vi "Classifier Utility.vi"() -> ()   [LabVIEW 2016]
uses:
  <vilib>/vision/Classification.llb/IMAQ SVM Kernel Options.ctl
  _vlib/CU_ClassifierQualityMeasure.ctl
  _vlib/CU_metaParameters.ctl
  _vlib/CU_metaIndicators.ctl
  Classifier.lvlib
  <vilib>/Analysis/NI_AALBase.lvlib
panel:
  in  "Stop Button":bool
  in  "Tab Control":T1(tab)
  in  "ClassifierQualityMeasure":T2 caption="Критерий оценки точности классификации"
  in  "Training data paths":path[](array[path]) caption="Пути к файлам с обучающими данными"
  in  "Test data paths":path[](array[path]) caption="Пути к файлам с тестовыми данными"
  in  "True labels for Test data":path[](array[path]) caption="Пути к файлам с метками классов (для тестовых данных)"
  in  "Start GA":bool
  in  "SVM ClassifierOptions":T3={"Kernel"=enum."Linear", "Degree"=3, "Gamma"=1.0, "Coefficient"=0.0, "Sigma"=1.0, "Cache(MB)"=200.0} caption="Настройки метода опорных векторов"
  in  "Pointer Slide":dbl(slide) caption="Сократить число признаков на %" min=0.0 max=100.0 step=1.0 scale=0.0..100.0
  in  "Use equal number of trials?":bool caption="Включить балансировку классов?"
  out "kNN accuracy":dbl caption="Макс. среднее\nзнач. точности"
  out "Best k value":dbl caption="Оптимальное\nзначение k"
  out "kNN classifier":cluster{dbl[], dbl[]}[](graph) caption="Метод k ближайших соседей"
  out "SVM classifier":cluster{dbl[], dbl[]}[](graph) caption="Метод опорных векторов"
  out "Best Nu value":dbl caption="Оптимальное \nзначение Nu"
  out "SVM accuracy":dbl caption="Макс. среднее\nзнач. точности"
  out "MLP accuracy":dbl caption="Макс. среднее\nзнач. точности"
  out "Best N value":dbl caption="Оптимальное\nзначение N"
  out "MLP classifier":cluster{dbl[], dbl[]}[](graph) caption="Многослойный персептрон"
  out "Dataset Num":i32
  out "Total Progress":i32(slide) scale=0.0..3.0
  out "Solution":i32(listbox) caption="Оценки точности классификации"
  out "Accuracies Graph":cluster{dbl[], dbl[]}[](graph) caption="Графики точности классификации"
  out "Results":string caption="Протокол выполнения программы"
  out "Accuracies out":dbl[][](array[numeric]) caption="Оценки точности классификации" format="%#_3g"
  out "Average  Accuracies":dbl[][](array[numeric]) caption="Точность классификации по всем наборам данных" format="%#_3g"
  # "This VI is a part of BCI Design library, http://www.ru-bci.org \nCopyright © 2020, Sotnikov Peter, All rights reserved. License: GNU GPLv3"
  # "Общее выполнение"
  # "Набор данных №"
  # "Выбор оптимальных параметров классификаторов"
  # "Методы классификации"
  # "Среднее\nпо наборам"
  # "Метод классификации"
  # "K1"
  # "K2"
  # "K3"
  # "K4"
  # "K5"
  # "Среднее значение"
  # "Среднеквадратич. отклонение"
  # "Максимальное значение"
  # "Минимальное значение"
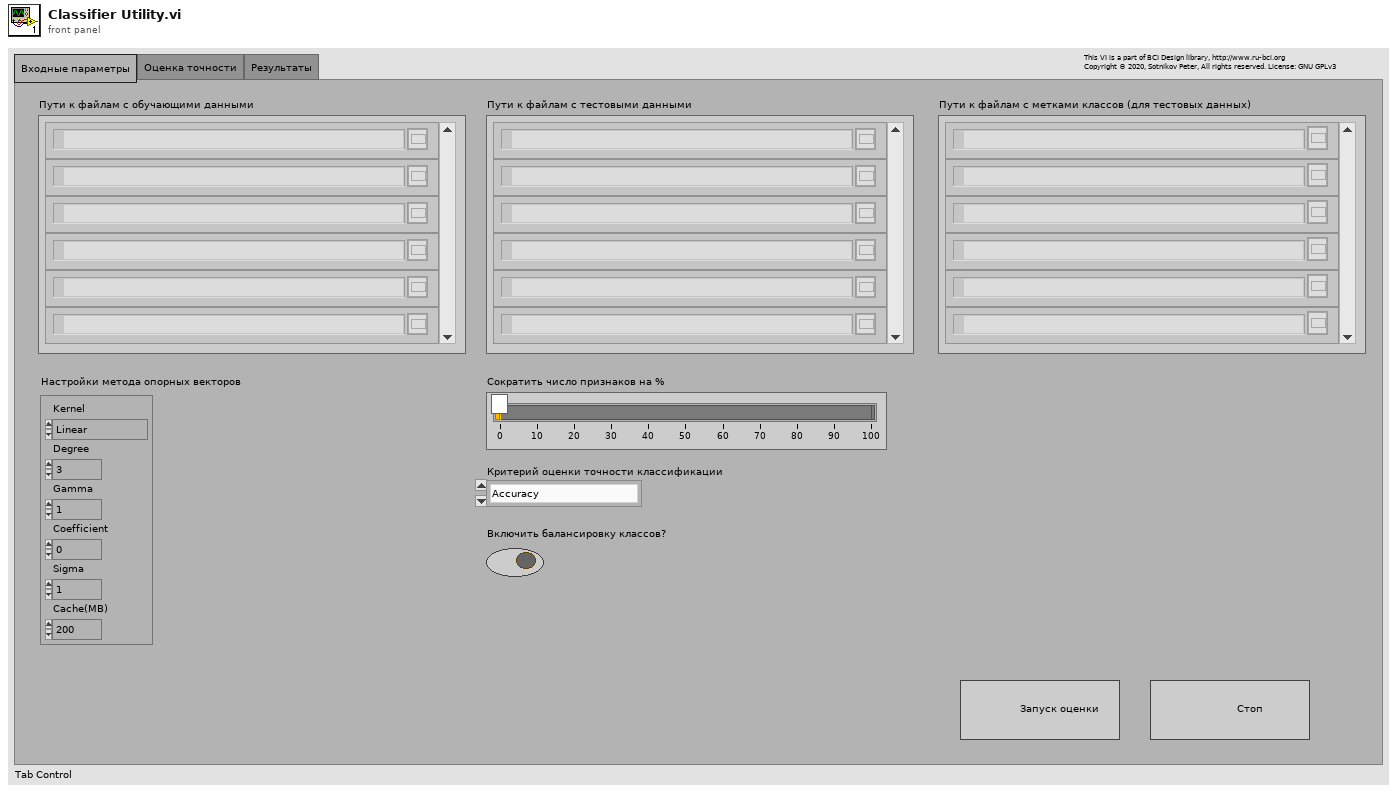
[diagram p1: front panel]
types:
  T1 = enum32{"Входные параметры", "Оценка точности", "Результаты"}
  T2 = typedef "Classifier.lvlib/CU_ClassifierQualityMeasure.ctl" = enum16{"Accuracy", "Cohen's kappa"}
  T3 = typedef "IMAQ SVM Kernel Options.ctl" = cluster{"Kernel":enum32{"Linear", "Polynomial", "Gaussian", "RBF"}, "Degree":i32, "Gamma":dbl, "Coefficient":dbl, "Sigma":dbl, "Cache(MB)":dbl}
  T4 = typedef "Classifier.lvlib/CU_metaIndicators.ctl" = cluster{"Accuracy Charts":refnum<vi>[], "Best Parameter Vals":refnum<vi>[], "Max Accuracies":refnum<vi>[]}
  T5 = typedef "Classifier.lvlib/CU_metaParameters.ctl" = cluster{"Training Data Path":path, "Test Data Path":path, "True Labels Path":path, "SVM ClassifierOptions":T3, "% of redundant features":dbl, "Use equal number of trials?":bool, "ClassifierQualityMeasure":T2}
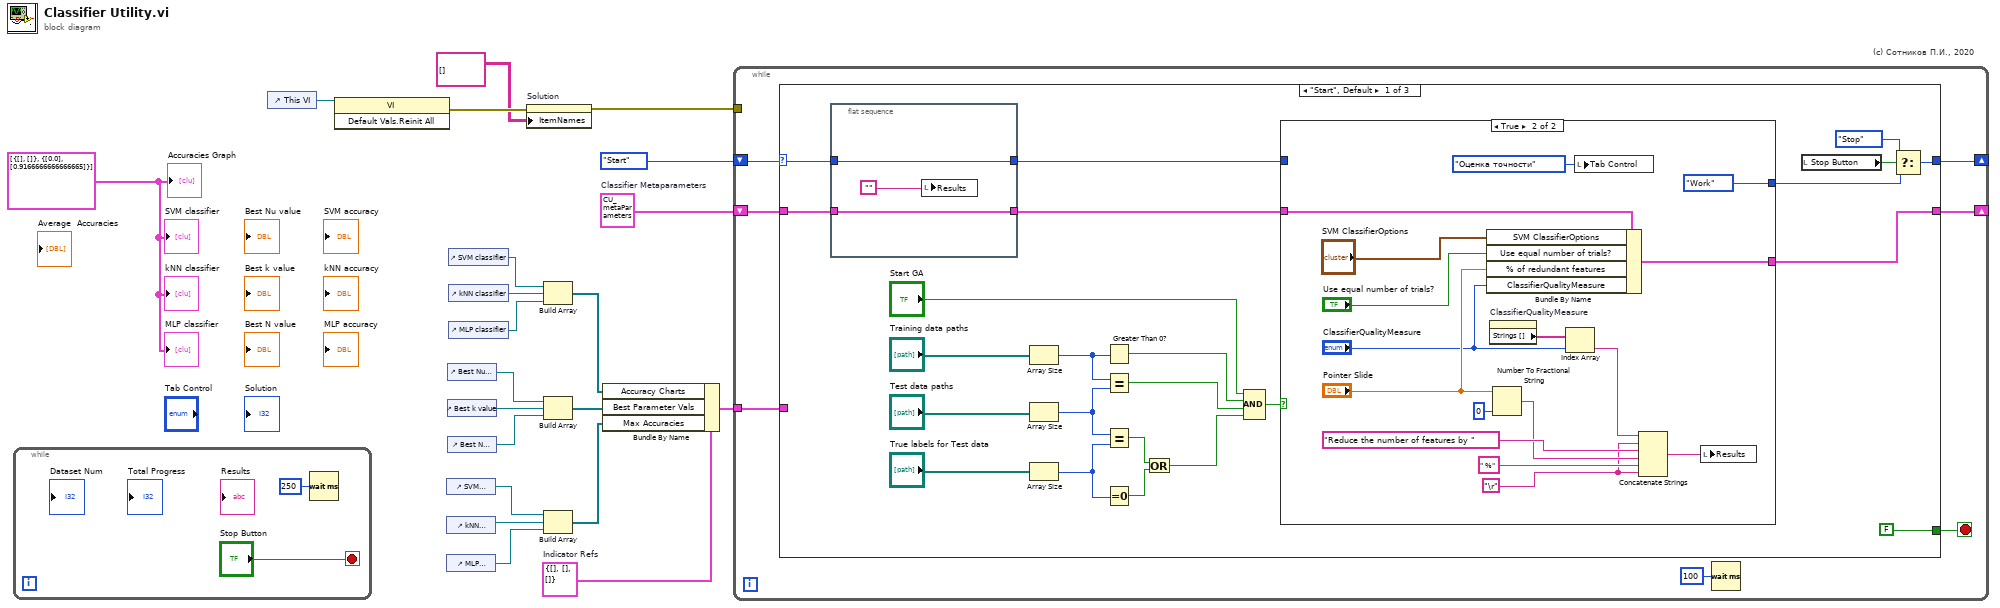
[diagram p0: block diagram]
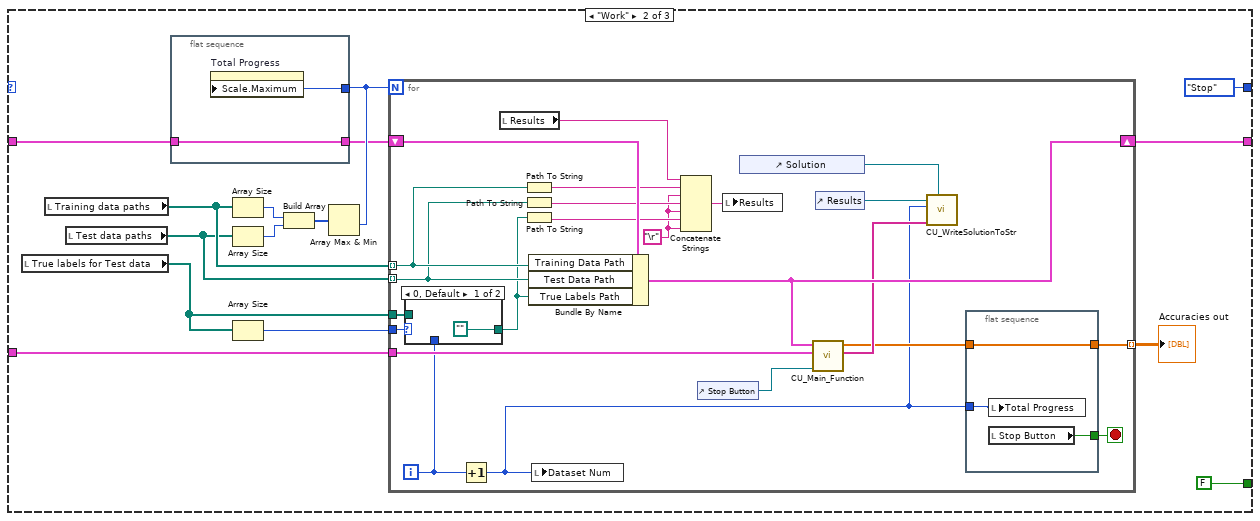
[diagram p3: hidden frame]
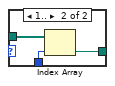
[diagram p4: hidden frame]
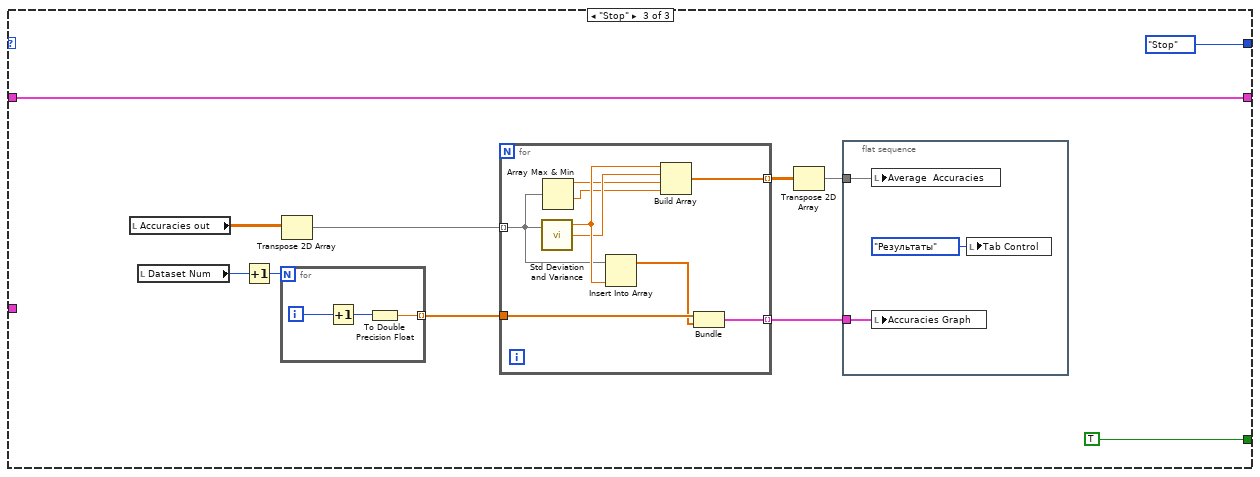
[diagram p5: hidden frame]
diagram:
  w1 = cluster{dbl[], dbl[]}[] [{[], []}, {[0.0], [0.9166666666666665]}] ("Accuracies Graph")
  w7 = T4 {"Accuracy Charts"=[], "Best Parameter Vals"=[], "Max Accuracies"=[]}  # Indicator Refs
  w17 = T5 {"Training Data Path"=path "", "Test Data Path"=path "", "True Labels Path"=path "", "SVM ClassifierOptions"={"Kernel"=enum."Linear", "Degree"=3, "Gamma"=1.0, "Coefficient"=0.0, "Sigma"=1.0, "Cache(MB)"=200.0}, "% of redundant features"=0.0, "Use equal number of trials?"=FALSE, "ClassifierQualityMeasure"=enum."Accuracy"}  # Classifier Metaparameters
  # "(с) Сотников П.И., 2020"
  n1 = while {
    stop <- "Stop Button" stop-if-true
    n2 = Wait (ms)(milliseconds to wait=u32 250) -> ()  [unwired: 1 out]
  }
  n3 = control-ref of="This VI"() -> (w20:refnum<vi>)
  n4 = invoke class="VI" method="Default Vals.Reinit All"(reference=w20) -> (error out=w19:errorcluster)  [unwired: 2 in, 2 out]
  n5 = control-ref of="SVM accuracy"() -> (w10:refnum<vi>)
  n6 = control-ref of="kNN accuracy"() -> (w9:refnum<vi>)
  n7 = control-ref of="MLP accuracy"() -> (w8:refnum<vi>)
  n8 = control-ref of="Best Nu value"() -> (w13:refnum<vi>)
  n9 = control-ref of="Best k value"() -> (w12:refnum<vi>)
  n10 = control-ref of="Best N value"() -> (w11:refnum<vi>)
  n11 = control-ref of="SVM classifier"() -> (w14:refnum<vi>)
  n12 = control-ref of="kNN classifier"() -> (w15:refnum<vi>)
  n13 = control-ref of="MLP classifier"() -> (w16:refnum<vi>)
  n14 = property on="Solution" class="MCListbox (strict)"(error in=w19, "ItemNames"=string[][] [] ("Item Names")) -> (error out=w2:errorcluster)  [unwired: 1 in, 1 out]
  n15 = Build Array(w14, w15, w16) -> (w5:refnum<vi>[])
  n16 = Build Array(w13, w12, w11) -> (w6:refnum<vi>[])
  n17 = Build Array(w10, w9, w8) -> (w4:refnum<vi>[])
  n18 = Bundle By Name(cluster=w7, "Accuracy Charts"=w5, "Best Parameter Vals"=w6, "Max Accuracies"=w4) -> (w3:T4)
  n19 = while {
    shift-right: [w27] -> _
    shift-left: w17 -> [w29]
    shift-right: [w28] -> _
    shift-left: enum16{"Start", "Work", "Stop"}."Start" -> [w30]
    tunnel: w3 -> [w24]
    tunnel: w2 -> [_]
    stop <- w25 stop-if-true
    n20 = case shown="\"Start\", Default" w30 {
      selector: w30 -> [w42 _ _]
      tunnel: w29 -> [w40 w75 w131]
      tunnel: [w45 enum16{"Start", "Work", "Stop"}."Stop" ("t") enum16{"Start", "Work", "Stop"}."Stop" ("t")] -> w28
      tunnel: [w47 w83 w131] -> w27
      tunnel: [FALSE FALSE TRUE] -> w25
      tunnel: w24 -> [_ w81 _]
      frame "Start", Default {
        n21 = flat-sequence {
          tunnel: w42 -> [w56]
          tunnel: [w56] -> w41
          tunnel: w40 -> [w55]
          tunnel: [w55] -> w39
          frame #0 {
            n22 = local write "Results"("") -> ()
          }
        }
        n23 = Array Size(array="Training data paths") -> (size(s)=w33:i32)
        n24 = Array Size(array="Test data paths") -> (size(s)=w53:i32)
        n25 = Array Size(array="True labels for Test data") -> (size(s)=w38:i32)
        n26 = Greater Than 0?(x=w33) -> (x > 0?=w32:bool)
        n27 = Equal?(x=w33, y=w53) -> (x = y?=w52:bool)
        n28 = Equal?(x=w53, y=w38) -> (x = y?=w36:bool)
        n29 = Equal To 0?(x=w38) -> (x = 0?=w37:bool)
        n30 = Or(x=w36, y=w37) -> (x .or. y?=w35:bool)
        n31 = Compound Arithmetic op=AND("Start GA", w32, w52, w35) -> (w51:bool)
        n32 = case shown="True" w51 {
          tunnel: w39 -> [w58 w74]
          tunnel: w41 -> [w57 _]
          tunnel: [w57 enum16{"Start", "Work", "Stop"}."Work"] -> w43
          tunnel: [w58 w73] -> w47
          frame False {
          }
          frame True {
            w59 = "\r"
            n33 = Bundle By Name(cluster=w74, "SVM ClassifierOptions"="SVM ClassifierOptions", "Use equal number of trials?"="Use equal number of trials?", "% of redundant features"="Pointer Slide", "ClassifierQualityMeasure"="ClassifierQualityMeasure") -> (w73:T5)
            n34 = property on="ClassifierQualityMeasure" class="Enum (strict)"() -> ("Strings []"=w62:string[])  [unwired: 2 in, 2 out]
            n35 = Number To Fractional String(number="Pointer Slide", precision (6)=i16 0) -> (F-format string=w68:string)  [unwired: 2 in]
            n36 = Index Array(array=w62, index="ClassifierQualityMeasure") -> (element=w60:string)
            n37 = local write "Tab Control"(T1."Оценка точности" ("Tab Control")) -> ()
            n38 = Concatenate Strings(w60, w59, "Reduce the number of features by " ("string"), w68, " %" ("string"), w59) -> (w72:string)
            n39 = local write "Results"(w72) -> ()
          }
        }
        n40 = local read "Stop Button"() -> (w44:bool)
        n41 = Select(t=enum16{"Start", "Work", "Stop"}."Stop", s=w44, f=w43) -> (s? t:f=w45:enum16{"Start", "Work", "Stop"})
      }
      frame "Work" {
        n42 = local read "True labels for Test data"() -> (w79:path[])
        n43 = local read "Training data paths"() -> (w85:path[])
        n44 = local read "Test data paths"() -> (w84:path[])
        n45 = flat-sequence {
          tunnel: w82 -> [w91]
          tunnel: [w90] -> w76
          tunnel: w75 -> [w90]
          frame #0 {
            n46 = property on="Total Progress" class="Slide (strict)"("Scale.Maximum"=w91) -> ()  [unwired: 2 in, 2 out]
          }
        }
        n47 = Array Size(array=w85) -> (size(s)=w88:i32)
        n48 = Array Size(array=w84) -> (size(s)=w87:i32)
        n49 = Array Size(array=w79) -> (size(s)=w78:i32)
        n50 = Build Array(w88, w87) -> (w86:i32[])
        n51 = Array Max & Min(array=w86) -> (min value=w82:i32)  [unwired: 3 out]
        n52 = for {
          N: w82 -> [_]
          tunnel: w85 -> [w108] mode=indexing
          tunnel: w84 -> [w107] mode=indexing
          tunnel: w79 -> [w95]
          shift-right: [w111] -> w83
          shift-left: w76 -> [w113]
          tunnel: w81 -> [w109]
          tunnel: [w97] -> w80 mode=indexing
          tunnel: w78 -> [w96]
          i -> [w94]
          stop <- w114 stop-if-true
          w102 = "\r"
          n53 = case shown="0, Default" w96 {
            tunnel: w95 -> [_ w118]
            tunnel: w94 -> [_ w117]
            tunnel: [path "" w116] -> w93
            frame 0, Default {
            }
            frame 1.. {
              n54 = Index Array(array=w118, index=w117) -> (element=w116:path)
            }
          }
          n55 = Increment(x=w94) -> (x+1=w92:i32)
          n56 = local read "Results"() -> (w106:string)
          n57 = Path To String(path=w108) -> (string=w105:string)
          n58 = Path To String(path=w107) -> (string=w104:string)
          n59 = Path To String(path=w93) -> (string=w103:string)
          n60 = Bundle By Name(cluster=w113, "Training Data Path"=w108, "Test Data Path"=w107, "True Labels Path"=w93) -> (w111:T5)
          n61 = local write "Dataset Num"(w92) -> ()
          n62 = Concatenate Strings(w106, w105, w102, w104, w102, w103, w102) -> (w101:string)
          n63 = control-ref of="Stop Button"() -> (w112:refnum<vi>)
          n64 = local write "Results"(w101) -> ()
          n65 = control-ref of="Solution"() -> (w99:refnum<vi>)
          n66 = call "CU_Main_Function.vi"("Stop Button Ref"=w112, "Indicator Refs in"=w109, "Classifier Metaparameters in"=w111) -> ("Accuracies String out"=w100:string[], "Accuracies out"=w98:dbl[])  [unwired: 7 in]
          n67 = control-ref of="Results"() -> (w110:refnum<vi>)
          n68 = call "CU_WriteSolutionToStr.vi"("ListBox Ref in"=w99, "Solution in"=w100, "Dataset Num"=w92, "String Ref in"=w110) -> ()  [unwired: 6 in, 2 out]
          n69 = flat-sequence {
            tunnel: [w121] -> w114
            tunnel: w98 -> [w120]
            tunnel: [w120] -> w97
            tunnel: w92 -> [w119]
            frame #0 {
              n70 = local write "Total Progress"(w119) -> ()
              n71 = local read "Stop Button"() -> (w121:bool)
            }
          }
        }
        "Accuracies out" <- w80
      }
      frame "Stop" {
        n72 = local read "Accuracies out"() -> (w130:dbl[][])
        n73 = local read "Dataset Num"() -> (w129:i32)
        n74 = Increment(x=w129) -> (x+1=w128:i32)
        n75 = for {
          N: w128 -> [_]
          tunnel: [w145] -> w126 mode=indexing
          i -> [w147]
          n76 = Increment(x=w147) -> (x+1=w146:i32)
          n77 = To Double Precision Float(number=w146) -> (double precision float=w145:dbl)
        }
        n78 = Transpose 2D Array(2D array=w130) -> (transposed array=w127:dbl[][])
        n79 = for {
          tunnel: w127 -> [w139] mode=indexing
          tunnel: w126 -> [w144]
          tunnel: [w142] -> w122 mode=indexing
          tunnel: [w136] -> w125 mode=indexing
          n80 = call <vilib>:"Std Deviation and Variance.vi"("X"=w139) -> ("mean"=w141:dbl, "standard deviation"=w140:dbl)  [unwired: 1 in, 1 out]
          n81 = Array Max & Min(array=w139) -> (max value=w138:dbl, min value=w137:dbl)  [unwired: 2 out]
          n82 = Insert Into Array(array=w139, new element=w141) -> (w143:dbl[])  [unwired: 1 in]
          n83 = Build Array(w141, w140, w138, w137) -> (w136:dbl[])
          n84 = Bundle(w144, w143) -> (w142:cluster{dbl[], dbl[]})  [unwired: 1 in]
        }
        n85 = Transpose 2D Array(2D array=w125) -> (transposed array=w124:dbl[][])
        n86 = flat-sequence {
          tunnel: w124 -> [w135]
          tunnel: w122 -> [w134]
          frame #0 {
            n87 = local write "Average  Accuracies"(w135) -> ()
            n88 = local write "Accuracies Graph"(w134) -> ()
            n89 = local write "Tab Control"(T1."Результаты" ("Tab Control")) -> ()
          }
        }
      }
    }
    n90 = Wait (ms)(milliseconds to wait=u32 100) -> ()  [unwired: 1 out]
  }
  "MLP classifier" <- w1
  "SVM classifier" <- w1
  "kNN classifier" <- w1
  "Accuracies Graph" <- w1
